vi "Read Compatible Hardware Types.vi"(8 "error in (no error)":errorcluster, 11 "Diode IV in":refnum<class "Diode IV.lvclass">) -> (0 "error out":errorcluster, 2 "Compatible Hardware Types":string[](array[string]), 3 "Diode IV out":refnum<class "Diode IV.lvclass">)   [LabVIEW 2013, in "Diode Characterization.lvlib" / "Diode IV.lvclass"]
uses:
  Diode IV.lvclass
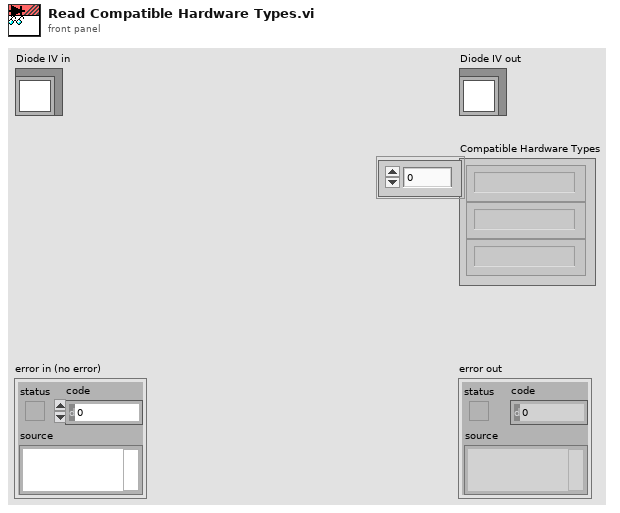
[diagram p1: front panel]
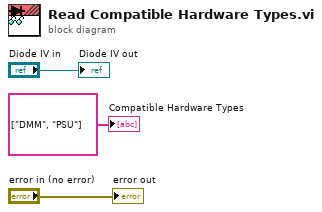
[diagram p0: block diagram]
diagram:
  "error out" <- "error in (no error)"
  "Diode IV out" <- "Diode IV in"
  "Compatible Hardware Types" <- string[] ["DMM", "PSU"] ("Compatible Hardware Types")
